vi "Auto Index.vi"(8 "error in (no error)":errorcluster, 11 "RelayValue":T1) -> (0 "error out":errorcluster)   [LabVIEW 2015]
uses:
  <vilib>/Rock Robotics/WPI/Relay/WPI_RelayValue.ctl
  Global Variables/Refnum Names.vi
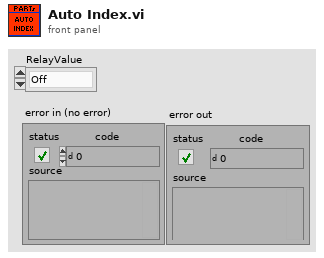
[diagram p1: front panel]
types:
  T1 = typedef "WPI_RelayValue.ctl" = enum16{"Off", "On", "Forward", "Reverse"}
  T2 = typedef "WPI_RelayDevRef.ctl" = cluster{"DevStatus":errorcluster, "Relay Channel":T3, "Relay Direction":T4}
  T3 = typedef "FPGA_DIORelayChannel.ctl" = enum8{"Relay 0", "Relay 1", "Relay 2", "Relay 3", "Invalid"}
  T4 = typedef "WPI_RelayDirection.ctl" = enum16{"Both directions", "Forward only", "Reverse only"}
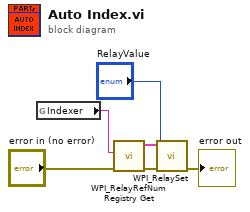
[diagram p0: block diagram]
diagram:
  n1 = global read "Refnum Names.vi" "Indexer"() -> (w6:string)
  n2 = call <vilib>:"WPI_RelayRefNum Registry Get.vi"("error in (no error)"="error in (no error)", "refnum name"=w6) -> ("error out"=w5:errorcluster, "RelayDevRef"=w4:T2)  [unwired: 8 in]
  n3 = call <vilib>:"WPI_RelaySet.vi"("error in (no error)"=w5, "RelayValue"="RelayValue", "RelayDevRef"=w4) -> ("error out"=→"error out":errorcluster)  [unwired: 7 in, 1 out]
